vi "Set DDS Loops Num Infinity.vi"(10 "en":i32, 11 "channel_index":u8) -> ()   [LabVIEW 2021, in "vmmso.lvlib"]
doc: "DLL_API void WINAPI SetDDSLoopsNumInfinity(unsigned char channel_index, int en);"
uses:
  vmmso.lvlib
  vmmso.dll
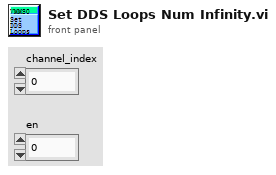
[diagram p1: front panel]
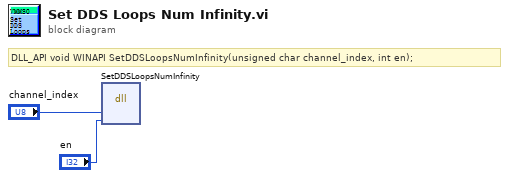
[diagram p0: block diagram]
diagram:
  # "DLL_API void WINAPI SetDDSLoopsNumInfinity(unsigned char channel_index, int en);"
  n1 = dll-call lib="D:/labviewdemo/LabviewDemo 21/vmmso/vmmso.*" fn="SetDDSLoopsNumInfinity"("channel_index"="channel_index", "en"="en") -> ()  [unwired: 6 in, 2 out]
